vi "Example To Variant.vi"() -> ()   [LabVIEW 2018]
uses:
  Transcriptors/System API/Basic Datatypes Pointers/CharPointer.lvclass
  Transcriptors/System API/Basic Datatypes Pointers/UnsignedCharPointer.lvclass
panel:
  out "data 3":sgl
  out "data 2":refnum<class "CharPointer.lvclass">[](array[class])
  out "data":refnum<class "CharPointer.lvclass">
  out "error out":errorcluster
  in  "error in":errorcluster
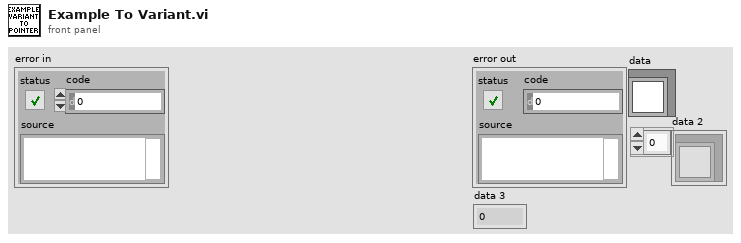
[diagram p1: front panel]
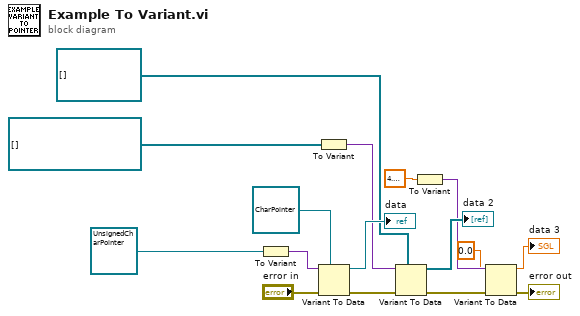
[diagram p0: block diagram]
diagram:
  n1 = To Variant(anything=refnum<class "UnsignedCharPointer.lvclass"> refnum ("UnsignedCharPointer.lvclass")) -> (Variant=w15:variant)
  n2 = To Variant(anything=refnum<class "UnsignedCharPointer.lvclass">[] []) -> (Variant=w10:variant)
  n3 = Variant To Data(error in="error in", type=refnum<class "CharPointer.lvclass"> refnum ("CharPointer.lvclass"), Variant=w15) -> (data=→"data":refnum<class "CharPointer.lvclass">, error out=w12:errorcluster)
  n4 = Variant To Data(error in=w12, type=refnum<class "CharPointer.lvclass">[] [], Variant=w10) -> (data=→"data 2":refnum<class "CharPointer.lvclass">[], error out=w6:errorcluster)
  n5 = To Variant(anything=sgl 4.2) -> (Variant=w4:variant)
  n6 = Variant To Data(error in=w6, type=sgl 0.0, Variant=w4) -> (data=→"data 3":sgl, error out=→"error out":errorcluster)
